vi "Number to string.vi"(8 "Error In":errorcluster, 11 "Integer":i32) -> (0 "Error Out":errorcluster, 3 "String":string)   [LabVIEW 2016]
doc: "Number to String VI converts control values to string adding 0 to ones that are less than 10."
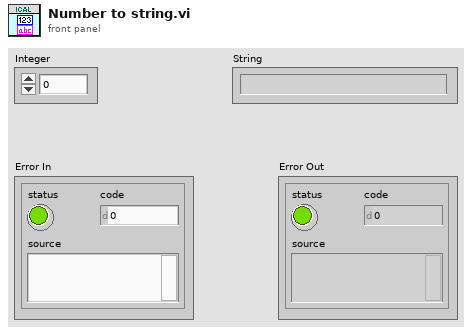
[diagram p1: front panel]
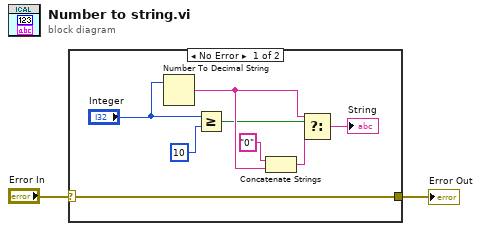
[diagram p0: block diagram]
diagram:
  n1 = case shown="No Error" "Error In" {
    selector: "Error In" -> [w3 w11]
    tunnel: [w3 w11] -> w1
    frame No Error {
      n2 = Number To Decimal String(number="Integer") -> (decimal integer string=w8:string)  [unwired: 1 in]
      n3 = Greater Or Equal?(x="Integer", y=10) -> (x >= y?=w5:bool)
      n4 = Concatenate Strings("0" ("string"), w8) -> (w9:string)
      n5 = Select(t=w8, s=w5, f=w9) -> (s? t:f=→"String":string)
    }
    frame Error {
    }
  }
  "Error Out" <- w1
